vi "subAxopatch_GenSealTestWave.vi"(8 "Error in (no error)":errorcluster, 11 "Pipet tuning parameters":T2={"Amplitude (mV)"=10.0, "Number of repeats"=20, "Sampling rate (Hz)"=20000.0, "Wave Freq. (Hz)"=10.0}) -> (0 "Error out":errorcluster, 3 "Patch seal test wavefrom":waveform(dbl)(graph)={"t0"=timestamp(0 s since 1904-01-01), "dt"=5e-05, "Y"=array[40000 elements]}, 5 "Seal test DAQ params":T1={"samples"=0, "Duration (sec)"=2.0, "Downsampling factor"=2000.0})   [LabVIEW 2015]
uses:
  <vilib>/measure/NI_MABase.lvlib
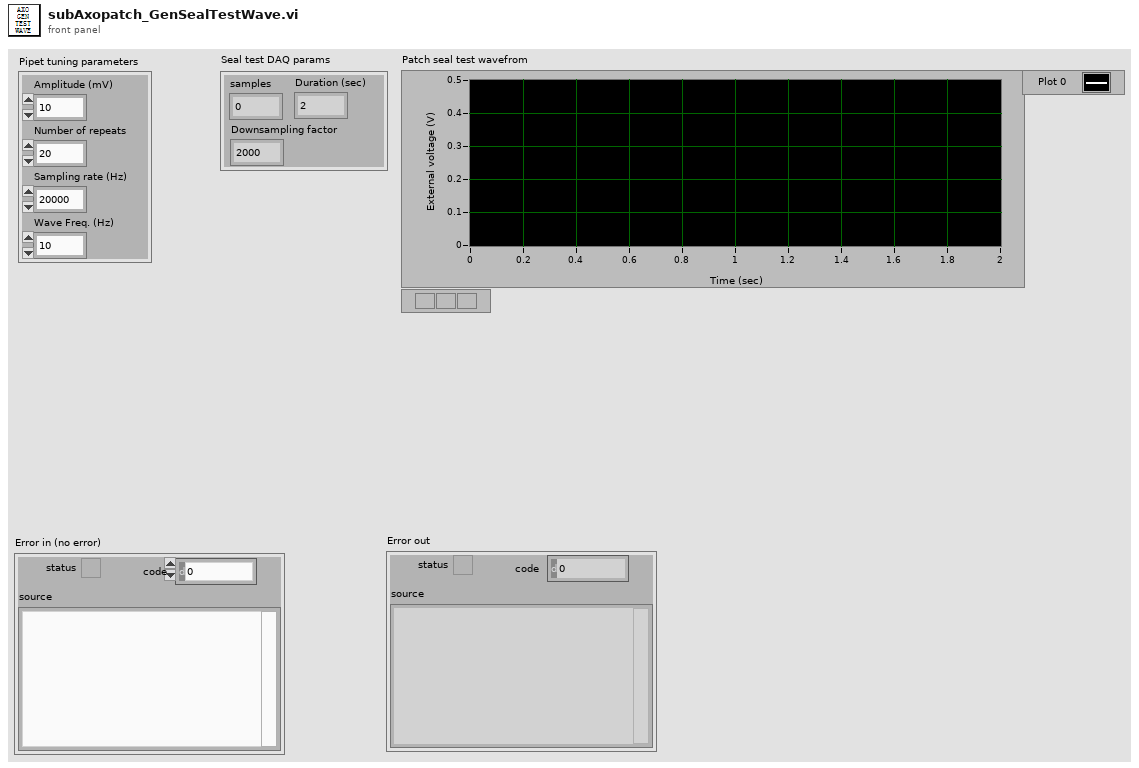
[diagram p1: front panel]
types:
  T1 = cluster{"samples":i32, "Duration (sec)":dbl, "Downsampling factor":dbl}
  T2 = cluster{"Amplitude (mV)":dbl, "Number of repeats":i32, "Sampling rate (Hz)":dbl, "Wave Freq. (Hz)":dbl}
  T3 = enum16{"Sine Wave", "Triangle Wave", "Square Wave", "Sawtooth Wave"}
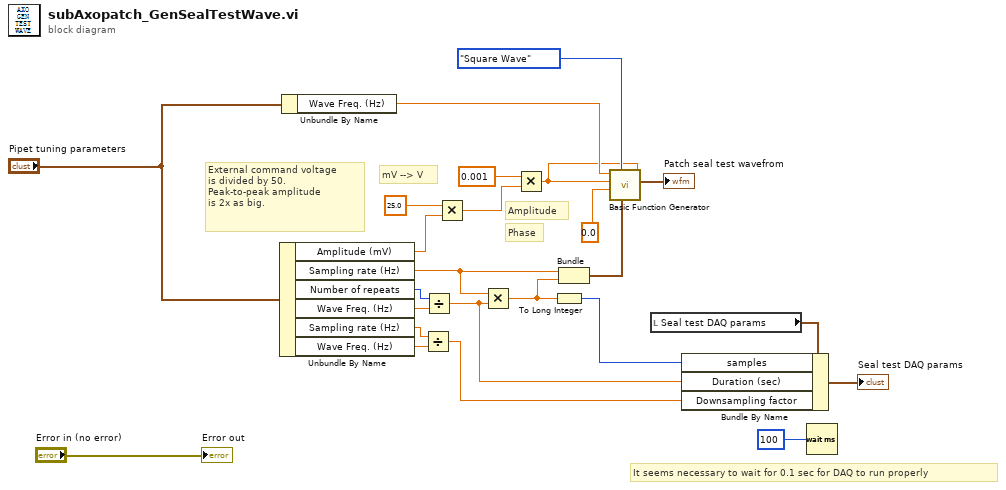
[diagram p0: block diagram]
diagram:
  # "Amplitude"
  # "It seems necessary to wait for 0.1 sec for DAQ to run properly"
  # "Phase"
  # "mV --> V"
  # "External command voltage\nis divided by 50. \nPeak-to-peak amplitude\nis 2x as big."
  n1 = Unbundle By Name("Pipet tuning parameters") -> ("Amplitude (mV)"=w23:dbl, "Sampling rate (Hz)"=w18:dbl, "Number of repeats"=w16:i32, "Wave Freq. (Hz)"=w17:dbl, "Sampling rate (Hz)"=w21:dbl, "Wave Freq. (Hz)"=w22:dbl)
  n2 = Unbundle By Name("Pipet tuning parameters") -> ("Wave Freq. (Hz)"=w24:dbl)
  n3 = Divide(x=w21, y=w22) -> (x/y=w3:dbl)
  n4 = Divide(x=w16, y=w17) -> (x/y=w4:dbl)
  n5 = Multiply(x=25.0, y=w23) -> (x*y=w9:dbl)
  n6 = Multiply(x=w18, y=w4) -> (x*y=w11:dbl)
  n7 = Multiply(x=0.001, y=w9) -> (x*y=w7:dbl)
  n8 = To Long Integer(number=w11) -> (32bit integer=w5:i32)
  n9 = Bundle("Sampling rate (Hz)"=w18, w11) -> (w19:cluster{"Sampling rate (Hz)":dbl, dbl})  [unwired: 1 in]
  n10 = call <vilib>:"Basic Function Generator.vi"("offset"=w7, "sampling info"=w19, "signal type"=T3."Square Wave", "phase"=0.0, "amplitude"=w7, "frequency"=w24) -> ("signal out"=→"Patch seal test wavefrom":waveform(dbl))  [unwired: 3 in, 2 out]
  n11 = local read "Seal test DAQ params"() -> (w1:T1)
  n12 = Bundle By Name(cluster=w1, "samples"=w5, "Duration (sec)"=w4, "Downsampling factor"=w3) -> (→"Seal test DAQ params":T1)
  n13 = Wait (ms)(milliseconds to wait=u32 100) -> ()  [unwired: 1 out]
  "Error out" <- "Error in (no error)"
